vi "Obtain Loop Notifiers.vi"(8 "error in (no error)":errorcluster, 11 "Create New":bool) -> (0 "error out":errorcluster, 3 "Loop Ctrl Notifiers Cluster":T1)   [LabVIEW 2015, in "Tool Interface.lvlib"]
uses:
  Tool Interface.lvlib
  _Loop Ctrl Notifiers Cluster--typedef.ctl
  _HS Data Stream Params Cluster--typedef.ctl
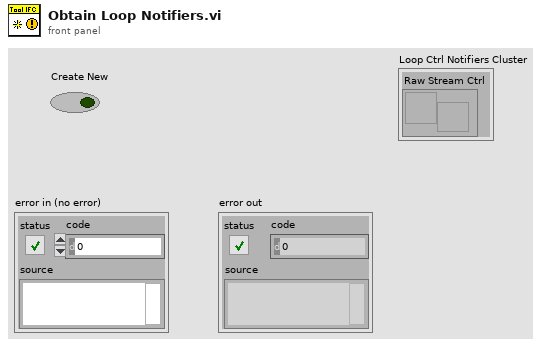
[diagram p1: front panel]
types:
  T1 = typedef "Tool Interface.lvlib/_Loop Ctrl Notifiers Cluster--typedef.ctl" = cluster{"Raw Stream Ctrl":refnum<notifier>}
  T2 = typedef "Tool Interface.lvlib/_HS Data Stream Params Cluster--typedef.ctl" = cluster{"Raw Data Stream Loop cmd":enum16{"Idle", "Receive HS Data", "Close Connection"}, "Data Array DVR ref":refnum<data-value>, "Sample Data notifier":refnum<notifier>, "Block Count Notifier":refnum<notifier>}
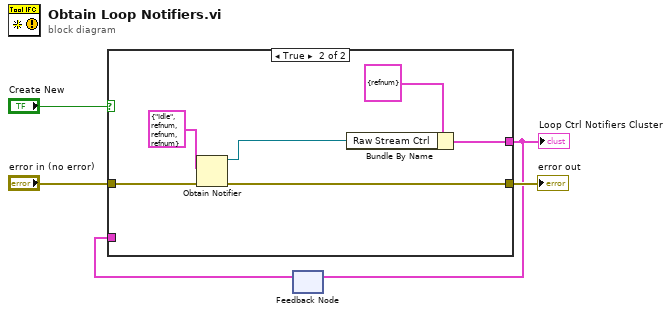
[diagram p0: block diagram]
diagram:
  n1 = feedback #1() -> (w1:T1)  [unwired: 1 in]
  n2 = case shown="True" "Create New" {
    tunnel: [w7 w12] -> w2
    tunnel: [w6 w8] -> w5
    tunnel: "error in (no error)" -> [w6 w11]
    tunnel: w1 -> [w7 _]
    frame False {
    }
    frame True {
      n3 = Obtain Notifier(notification data type=T2 {"Raw Data Stream Loop cmd"=enum."Idle", "Data Array DVR ref"=refnum, "Sample Data notifier"=refnum, "Block Count Notifier"=refnum} ("Cluster"), error in (no error)=w11) -> (notifier out=w9:refnum<notifier>, error out=w8:errorcluster)  [unwired: 2 in, 1 out]
      n4 = Bundle By Name(cluster=T1 {"Raw Stream Ctrl"=refnum} ("_Loop Ctrl Notifiers Cluster--typedef"), "Raw Stream Ctrl"=w9) -> (w12:T1)
    }
  }
  "error out" <- w5
  "Loop Ctrl Notifiers Cluster" <- w2
  n5 = feedback-in #1(w2) -> ()
